vi "Write Connection ID.vi"(8 "error in (no error)":errorcluster, 10 "Connection ID":refnum<k5>, 11 "RawSocket Handler in":refnum<class "RawSocket TCP Handler.lvclass">) -> (0 "error out":errorcluster, 3 "RawSocket Handler out":refnum<class "RawSocket TCP Handler.lvclass">)   [LabVIEW 2021, in "wamplv.lvlib" / "RawSocket TCP Handler.lvclass"]
uses:
  RawSocket TCP Handler.lvclass
  RawSocket TCP Handler.lvclass/RawSocket TCP Handler.ctl
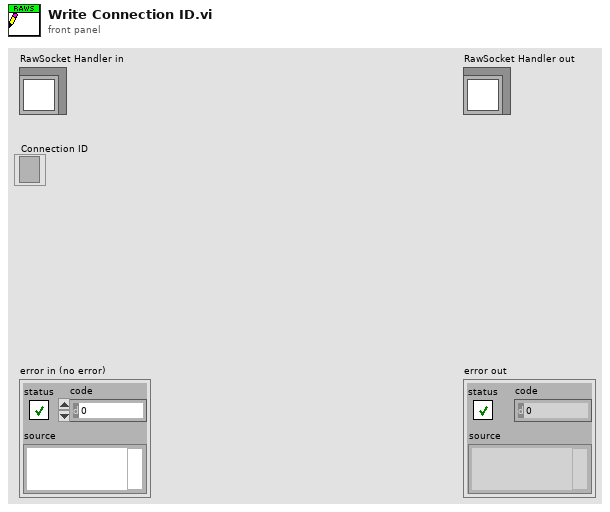
[diagram p1: front panel]
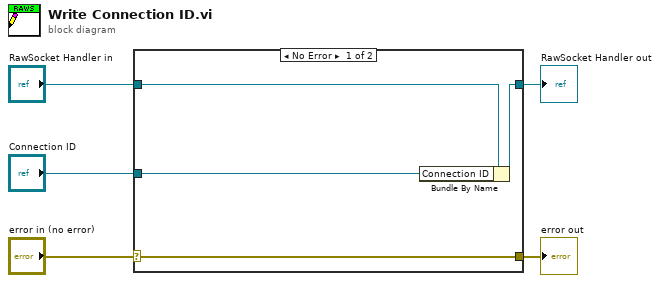
[diagram p0: block diagram]
diagram:
  n1 = case shown="No Error" "error in (no error)" {
    selector: "error in (no error)" -> [w9 w10]
    tunnel: [w9 w10] -> w4
    tunnel: [w7 w11] -> w2
    tunnel: "RawSocket Handler in" -> [w8 w11]
    tunnel: "Connection ID" -> [w6 _]
    frame No Error {
      n2 = Bundle By Name(cluster=w8, "Connection ID"=w6) -> (w7:refnum<class "RawSocket TCP Handler.lvclass">)
    }
    frame Error {
    }
  }
  "error out" <- w4
  "RawSocket Handler out" <- w2
